vi "Triax320 SetTurretPos.vi"(8 "error in (no error)":errorcluster, 10 "Grating":u8(ring) items=["1", "2", "3"], 11 "Triax VISA Rsrc":refnum<visa-resource-name>="SR530") -> (0 "error out":errorcluster, 2 "Grating Out":u8(ring) items=["1", "2", "3"], 3 "Triax VISA Rsrc Out":refnum<visa-resource-name>="SR530")   [LabVIEW 2019]
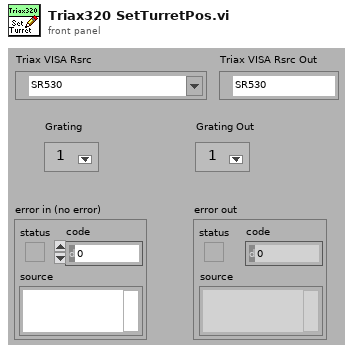
[diagram p1: front panel]
types:
  T1 = enum16{"Error", "Set Postion", "Wait Done", "Read Pos"}
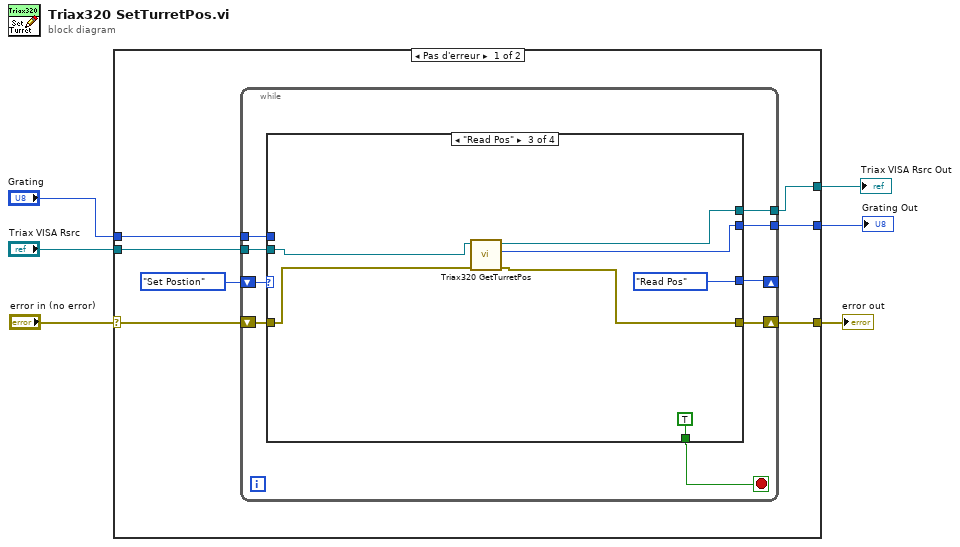
[diagram p0: block diagram]
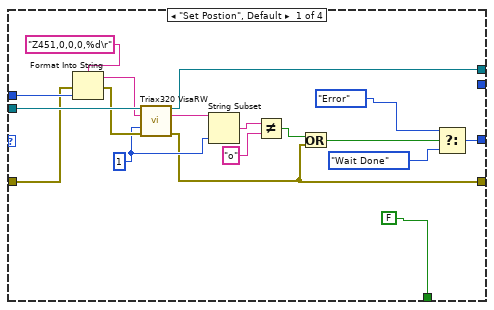
[diagram p2: hidden frame]
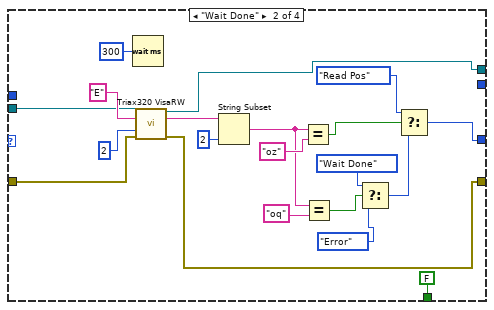
[diagram p3: hidden frame]
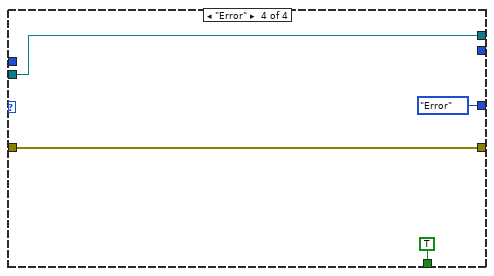
[diagram p4: hidden frame]
diagram:
  n1 = case shown="Pas d'erreur" "error in (no error)" {
    selector: "error in (no error)" -> [w12 w73]
    tunnel: "Triax VISA Rsrc" -> [w13 w72]
    tunnel: [w10 w73] -> w4
    tunnel: [w9 _] -> w2
    tunnel: [w8 w72] -> w3
    tunnel: "Grating" -> [w7 _]
    frame No Error {
      n2 = while {
        shift-right: [w20] -> _
        shift-left: T1."Set Postion" -> [w22]
        tunnel: w13 -> [w19]
        shift-right: [w17] -> w10
        shift-left: w12 -> [w18]
        tunnel: [w16] -> w8
        tunnel: [w15] -> w9
        tunnel: w7 -> [w14]
        stop <- w21 stop-if-true
        n3 = case shown="\"Read Pos\"" w22 {
          tunnel: [FALSE FALSE TRUE TRUE] -> w21
          tunnel: [w38 w44 T1."Read Pos" T1."Error"] -> w20
          tunnel: w19 -> [w40 w51 w67 w71]
          tunnel: w18 -> [w34 w52 w66 w69]
          tunnel: [w26 w42 w61 w69] -> w17
          tunnel: [w39 w43 w65 w71] -> w16
          tunnel: [_ _ w64 _] -> w15
          tunnel: w14 -> [w35 _ _ _]
          frame "Set Postion", Default {
            w30 = u32 1 ("Nbcaract")
            n4 = Format Into String(format string="Z451,0,0,0,%d\r" ("chaîne"), error in=w34, w35) -> (resulting string=w32:string, error out=w33:errorcluster)  [unwired: 1 in]
            n5 = call <userlib>:"Triax320 VisaRW.vi"("VISA Rsrc"=w40, "ChaineCom"=w32, "Nbcaract"=w30, "error in (no error)"=w33) -> ("VISA Rsrc Out"=w39:refnum<visa-resource-name>, "ChaineRep"=w31:string, "error out"=w26:errorcluster)  [unwired: 6 in, 3 out]
            n6 = String Subset(string=w31, length (rest)=w30) -> (substring=w29:string)  [unwired: 1 in]
            n7 = Not Equal?(x=w29, y="o" ("chaîne de format")) -> (x != y?=w27:bool)
            n8 = Or(x=w27, y=w26) -> (x .or. y?=w25:bool)
            n9 = Select(t=T1."Error", s=w25, f=T1."Wait Done") -> (s? t:f=w38:T1)
          }
          frame "Wait Done" {
            n10 = Wait (ms)(milliseconds to wait=u32 300 ("attente (ms)")) -> ()  [unwired: 1 out]
            n11 = call <userlib>:"Triax320 VisaRW.vi"("VISA Rsrc"=w51, "ChaineCom"="E" ("chaîne"), "Nbcaract"=u32 2, "error in (no error)"=w52) -> ("VISA Rsrc Out"=w43:refnum<visa-resource-name>, "ChaineRep"=w60:string, "error out"=w42:errorcluster)  [unwired: 6 in, 3 out]
            n12 = String Subset(string=w60, length (rest)=2 ("longueur (reste)")) -> (substring=w54:string)  [unwired: 1 in]
            n13 = Equal?(x=w54, y="oz") -> (x = y?=w47:bool)
            n14 = Equal?(x=w54, y="oq") -> (x = y?=w50:bool)
            n15 = Select(t=T1."Wait Done", s=w50, f=T1."Error") -> (s? t:f=w45:T1)
            n16 = Select(t=T1."Read Pos", s=w47, f=w45) -> (s? t:f=w44:T1)
          }
          frame "Read Pos" {
            n17 = call <userlib>:"Triax320 GetTurretPos.vi"("error in (no error)"=w66, "Triax VISA Rsrc"=w67) -> ("error out"=w61:errorcluster, "Grating"=w64:u8, "Triax VISA Rsrc Out"=w65:refnum<visa-resource-name>)  [unwired: 7 in]
          }
          frame "Error" {
          }
        }
      }
    }
    frame Error {
    }
  }
  "error out" <- w4
  "Triax VISA Rsrc Out" <- w3
  "Grating Out" <- w2
